vi "Generate Trig pulse_adv.vi"() -> ()   [LabVIEW 2020]
uses:
  <vilib>/eio/EIONode/EIONode.xnode
  <vilib>/rvi/eio/common/nirviEmuTemplateMethod_errors.vi
panel:
  in  "stop_train":bool
  in  "Pulse Width (us)":u32=100
  in  "Pulse Period (us)":u32=1000
  in  "Trigger Type":enum16{"Single Trigger", "Continuous Trigger"}(ring)
  in  "TL Input":bool
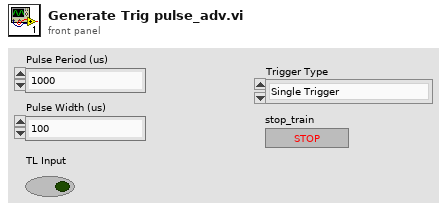
[diagram p1: front panel]
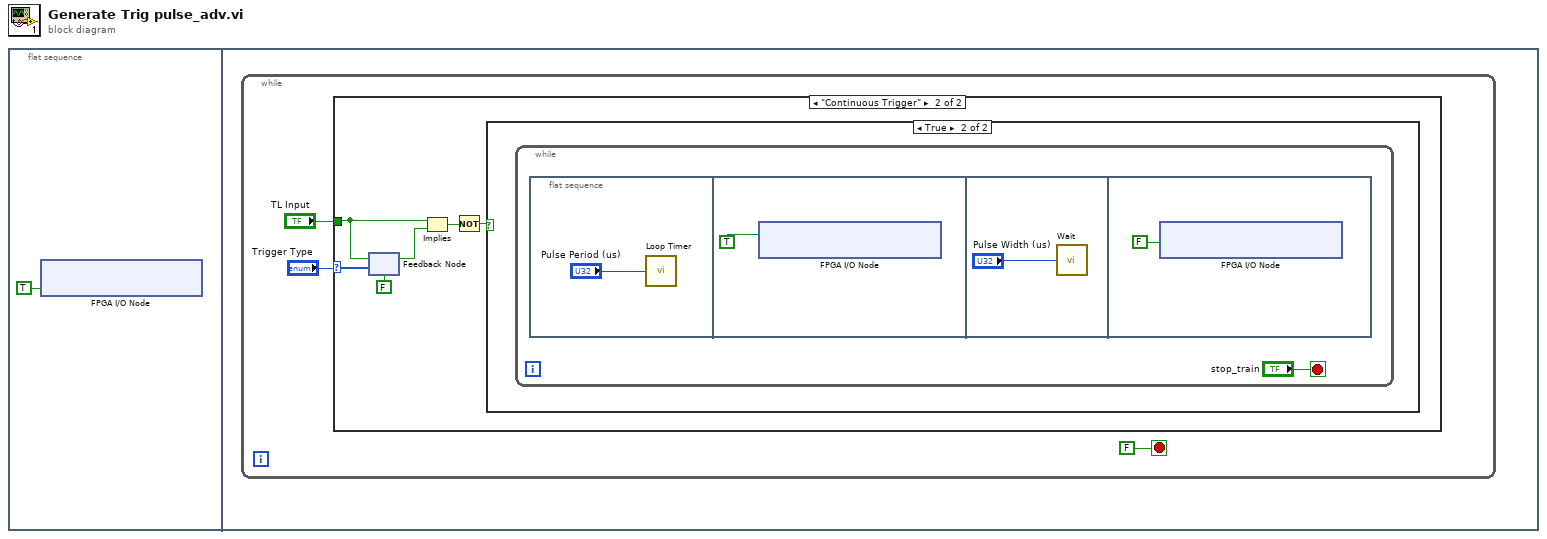
[diagram p0: block diagram]
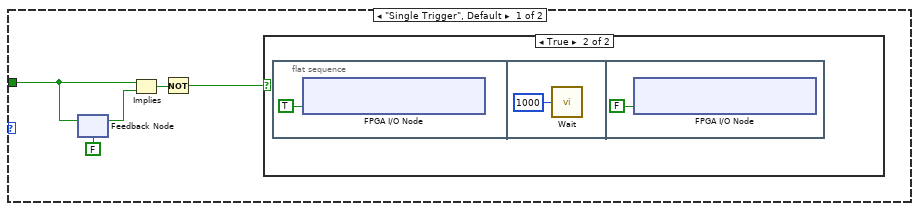
[diagram p2: hidden frame]
diagram:
  n1 = flat-sequence {
    frame #0 {
      n2 = xnode "FPGA I/O Node"("IO Module\\Trigger WE"=TRUE ("IO Module\\Trigger WE")) -> ()  [unwired: 1 in, 1 out]
    }
    frame #1 {
      n3 = while {
        stop <- FALSE stop-if-true
        n4 = case shown="\"Continuous Trigger\"" "Trigger Type" {
          tunnel: "TL Input" -> [w6 w14]
          frame "Single Trigger", Default {
            n5 = feedback #1(FALSE ("OK Button")) -> (w8:bool)
            n6 = feedback-in #1(w6) -> ()
            n7 = Implies(1:w8, 2:w6) -> (0:w9:bool)
            n8 = Not(x=w9) -> (.not. x?=w5:bool)
            n9 = case shown="True" w5 {
              frame False {
              }
              frame True {
                n10 = flat-sequence {
                  frame #0 {
                    n11 = xnode "FPGA I/O Node"("IO Module\\Trigger Output"=TRUE ("IO Module\\Trigger Output")) -> ()  [unwired: 1 in, 1 out]
                  }
                  frame #1 {
                    n12 = call "Wait"("Count(uSec)"=u32 1000 ("Count(mSec)")) -> ()  [unwired: 1 out]
                  }
                  frame #2 {
                    n13 = xnode "FPGA I/O Node"("IO Module\\Trigger Output"=FALSE ("IO Module\\Trigger Output")) -> ()  [unwired: 1 in, 1 out]
                  }
                }
              }
            }
          }
          frame "Continuous Trigger" {
            n14 = feedback #2(FALSE ("OK Button")) -> (w16:bool)
            n15 = feedback-in #2(w14) -> ()
            n16 = Implies(1:w16, 2:w14) -> (0:w17:bool)
            n17 = Not(x=w17) -> (.not. x?=w13:bool)
            n18 = case shown="True" w13 {
              frame False {
              }
              frame True {
                n19 = while {
                  stop <- "stop_train" stop-if-true
                  n20 = flat-sequence {
                    frame #0 {
                      n21 = call "Loop Timer"("Count(uSec)"="Pulse Period (us)") -> ()  [unwired: 1 out]
                    }
                    frame #1 {
                      n22 = xnode "FPGA I/O Node"("IO Module\\Trigger Output"=TRUE) -> ()  [unwired: 1 in, 1 out]
                    }
                    frame #2 {
                      n23 = call "Wait"("Count(uSec)"="Pulse Width (us)") -> ()  [unwired: 1 out]
                    }
                    frame #3 {
                      n24 = xnode "FPGA I/O Node"("IO Module\\Trigger Output"=FALSE) -> ()  [unwired: 1 in, 1 out]
                    }
                  }
                }
              }
            }
          }
        }
      }
    }
  }
